vi "SAVE_DATA.vi"(0 "Q_Process_Data_IN":refnum<queue>, 1 "Q_Process_Data_Err_IN":errorcluster, 2 "Q_SEND_IN":refnum<queue>, 3 "Q_SEND_Err_IN":errorcluster, 4 "Notifier_IN":refnum<notifier>, 5 "Notifier_Error_IN":errorcluster, 6 "Q_Process_Data2_IN":refnum<queue>, 8 "Q_Process_Data2_Err_IN":errorcluster caption="error out") -> (16 "Q_SEND_OUT":refnum<queue>, 17 "Q_SEND_Err_OUT":errorcluster)   [LabVIEW 2019]
uses:
  <vilib>/Platform/TimedLoop/XDataNode/timing_clust.ctl
  <vilib>/Platform/TimedLoop/XDataNode/nitl_modes.ctl
  <vilib>/Platform/TimedLoop/XDataNode/wakeup.ctl
  Type/Type_TCP_Cmd.ctl
  RT_GLOBAL.vi
  <vilib>/Platform/TimedLoop/XDataNode/XDataNode.xnode
  <vilib>/Platform/TimedLoop/XDataNode/XDNodeRunTimeDep.lvlib
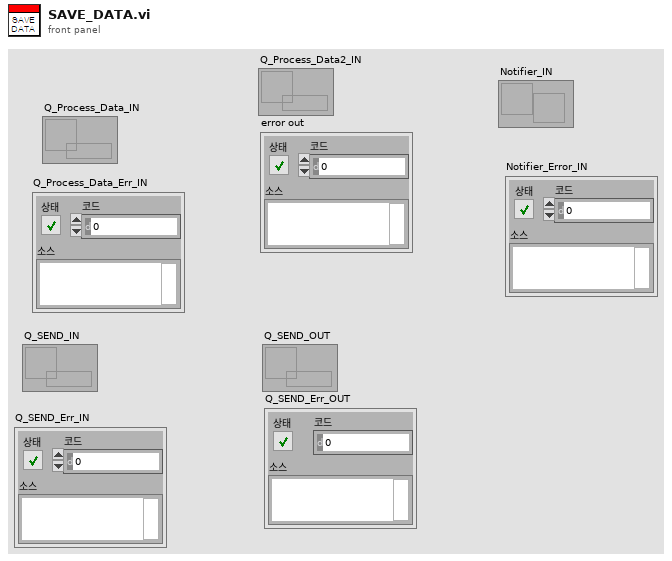
[diagram p1: front panel]
types:
  T1 = cluster{"Num_L":u32, "Period_L":u32, "GCP_L":sgl, "Num_R":u32, "Period_R":u32, "GCP_R":sgl, "FPGA_Data":sgl[], "Status_L":cluster{"Ready to switch on":bool, "Switched on":bool, "Operation enable":bool, "Fault":bool, "Voltage enable":bool, "Quick stop":bool, "Switch on disable":bool, "not used (warning)":bool, "Offset current measured":bool, "Remote":bool, "Operation mode specific":bool, "Internal limit active":bool, "Operation mode specific":bool, "Operation mode specific":bool, "Refresh cycle of power stage":bool, "Position referenced to home position":bool}, "Status_R":cluster{"Ready to switch on":bool, "Switched on":bool, "Operation enable":bool, "Fault":bool, "Voltage enable":bool, "Quick stop":bool, "Switch on disable":bool, "not used (warning)":bool, "Offset current measured":bool, "Remote":bool, "Operation mode specific":bool, "Internal limit active":bool, "Operation mode specific":bool, "Operation mode specific":bool, "Refresh cycle of power stage":bool, "Position referenced to home position":bool}, "Pos_L":i32, "Pos_R":i32, "TargetPos_L":i32, "TargetPos_R":i32, "Flag_L":enum16{"Release_Start", "Onset_Start", "Peak_Start", "Calculate"}, "Flag_R":enum16{"Release_Start", "Onset_Start", "Peak_Start", "Calculate"}, "LOAD_CELL_PEAK_L":sgl[], "LOAD_CELL_PEAK_R":sgl[], "D_Pos_L":i32, "D_Pos_R":i32, "A_Velocity_L":i32, "A_Velocity_R":i32, "A_Current_L":i16, "A_Current_R":i16}
  T2 = cluster{"Num_L":u32, "Period_L":u32, "GCP_L":sgl, "Num_R":u32, "Period_R":u32, "GCP_R":sgl, "FPGA_Data":sgl[], "Status_L":cluster{"Ready to switch on":bool, "Switched on":bool, "Operation enable":bool, "Fault":bool, "Voltage enable":bool, "Quick stop":bool, "Switch on disable":bool, "not used (warning)":bool, "Offset current measured":bool, "Remote":bool, "Operation mode specific":bool, "Internal limit active":bool, "Operation mode specific":bool, "Operation mode specific":bool, "Refresh cycle of power stage":bool, "Position referenced to home position":bool}, "Status_R":cluster{"Ready to switch on":bool, "Switched on":bool, "Operation enable":bool, "Fault":bool, "Voltage enable":bool, "Quick stop":bool, "Switch on disable":bool, "not used (warning)":bool, "Offset current measured":bool, "Remote":bool, "Operation mode specific":bool, "Internal limit active":bool, "Operation mode specific":bool, "Operation mode specific":bool, "Refresh cycle of power stage":bool, "Position referenced to home position":bool}, "Pos_L":i32, "Pos_R":i32, "TargetPos_L":i32, "TargetPos_R":i32, "Flag_L":enum16{"Release_Start", "Onset_Start", "Peak_Start", "Calculate"}, "Flag_R":enum16{"Release_Start", "Onset_Start", "Peak_Start", "Calculate"}, "LOAD_CELL_PEAK_L":sgl[], "LOAD_CELL_PEAK_R":sgl[], "D_Pos_L":i32, "D_Pos_R":i32, "A_Velocity_L":i32, "A_Velocity_R":i32, "A_Current_L":i16, "A_Current_R":i16}[]
  T3 = typedef "XDNodeRunTimeDep.lvlib/timing_clust.ctl" = cluster{"Expected End [f-1]":u64, "Actual End [f-1]":u64, "Finished Late? [f-1]":bool, "Expected End [i-1]":u64, "Actual End [i-1]":u64, "Finished Late? [i-1]":bool, "Expected Start [i]":u64, "Actual Start [i]":u64, "Expected Start [f]":u64, "Actual Start [f]":u64, "Source Name":string, "Structure Name":string, "Period":i64, "Deadline":i64, "Offset":i64, "Start":i64, "Priority":i32, "Timeout":i32, "Mode":T4, "Wakeup Reason":T5, "Error":errorcluster, "Source Type":string, "Secondary Source Type":string, "Global End Time":u64, "Global Start Time":u64, "Frame Duration":u64, "Iteration Duration":u64, "Assigned CPU":i32, "I/O Scan Engine Mode":u32}
  T4 = typedef "XDNodeRunTimeDep.lvlib/nitl_modes.ctl" = enum32{"No Change", "Process missed periods, maintain original phase", "Discard missed periods, maintain original phase", "Process missed periods, ignore original phase", "Discard missed periods, ignore original phase"}
  T5 = typedef "XDNodeRunTimeDep.lvlib/wakeup.ctl" = enum32{"Normal", "Aborted", "Asynchronous wakeup", "Timing source error", "Timed loop error", "Timeout"}
  T6 = typedef "Type_TCP_Cmd.ctl" = enum16{"None", "Data", "Config", "Active"}
  T7 = enum16{"open", "replace", "create", "open or create", "replace or create", "replace or create with confirmation"}
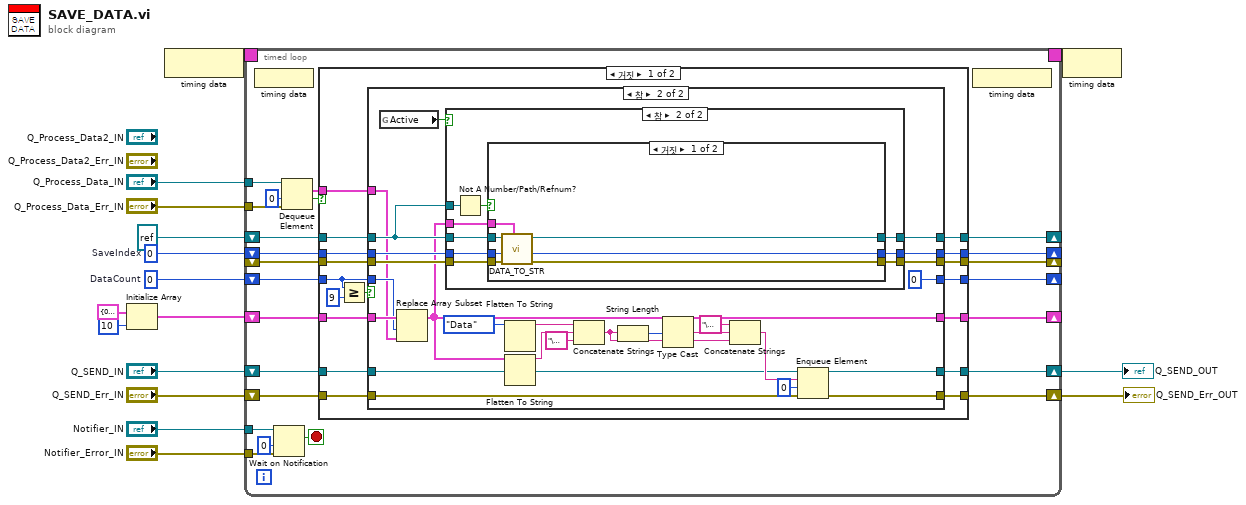
[diagram p0: block diagram]
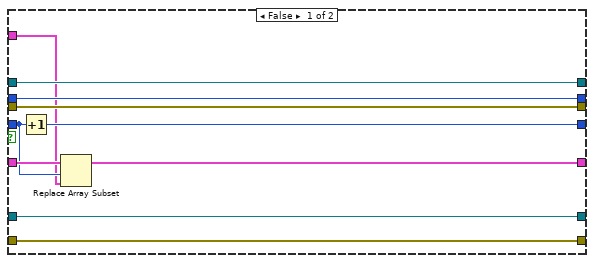
[diagram p2: hidden frame]
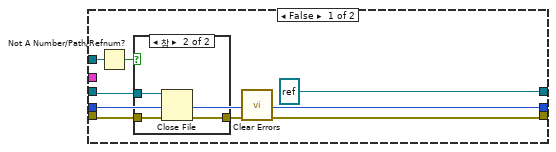
[diagram p3: hidden frame]
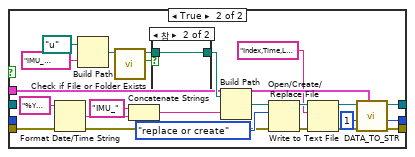
[diagram p5: hidden frame]
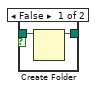
[diagram p6: hidden frame]
diagram:
  w14 = 0  # DataCount
  w15 = u32 0  # SaveIndex
  n1 = Initialize Array(T1 {"Num_L"=0, "Period_L"=0, "GCP_L"=0.0, "Num_R"=0, "Period_R"=0, "GCP_R"=0.0, "FPGA_Data"=[], "Status_L"={"Ready to switch on"=TRUE, "Switched on"=TRUE, "Operation enable"=TRUE, "Fault"=FALSE, "Voltage enable"=TRUE, "Quick stop"=TRUE, "Switch on disable"=FALSE, "not used (warning)"=FALSE, "Offset current measured"=FALSE, "Remote"=TRUE, "Operation mode specific"=TRUE, "Internal limit active"=FALSE, "Operation mode specific"=FALSE, "Operation mode specific"=FALSE, "Refresh cycle of power stage"=FALSE, "Position referenced to home position"=FALSE}, "Status_R"={"Ready to switch on"=TRUE, "Switched on"=TRUE, "Operation enable"=TRUE, "Fault"=FALSE, "Voltage enable"=TRUE, "Quick stop"=TRUE, "Switch on disable"=FALSE, "not used (warning)"=FALSE, "Offset current measured"=FALSE, "Remote"=TRUE, "Operation mode specific"=TRUE, "Internal limit active"=FALSE, "Operation mode specific"=FALSE, "Operation mode specific"=FALSE, "Refresh cycle of power stage"=FALSE, "Position referenced to home position"=FALSE}, "Pos_L"=0, "Pos_R"=0, "TargetPos_L"=0, "TargetPos_R"=0, "Flag_L"=enum."Release_Start", "Flag_R"=enum."Release_Start", "LOAD_CELL_PEAK_L"=[12.0, 8.0], "LOAD_CELL_PEAK_R"=[], "D_Pos_L"=0, "D_Pos_R"=0, "A_Velocity_L"=0, "A_Velocity_R"=0, "A_Current_L"=0, "A_Current_R"=0}, 10 ("차원 크기")) -> (w13:T2)
  n2 = node-c288() -> (w5:T3)
  n3 = timed-loop {
    tunnel: "Q_Process_Data_IN" -> [w38]
    tunnel: "Q_Process_Data_Err_IN" -> [w37]
    shift-right: [w34] -> _
    shift-left: refnum<file> refnum ("참조 번호 출력") -> [w35]
    shift-right: [w32] -> _
    shift-left: _ -> [w33]
    shift-right: [w31] -> _
    shift-left: w15 -> [w30]
    shift-right: [w28] -> _
    shift-left: w14 -> [w29]
    shift-right: [w26] -> _
    shift-left: w13 -> [w27]
    shift-right: [w24] -> w11
    shift-left: "Q_SEND_IN" -> [w25]
    shift-right: [w22] -> w10
    shift-left: "Q_SEND_Err_IN" -> [w23]
    timing: w5 -> [_]
    timing-out: [_] -> w4
    tunnel: "Notifier_IN" -> [w19]
    tunnel: "Notifier_Error_IN" -> [w18]
    stop <- w17 stop-if-true
    n4 = node-c288() -> ()  [unwired: 1 in]
    n5 = Wait on Notification(notifier=w19, timeout in ms (-1)=0 ("타임아웃(ms) (-1)"), error in (no error)=w18) -> (notification=w17:bool)  [unwired: 1 in, 3 out]
    n6 = Dequeue Element(queue=w38, timeout in ms (-1)=0 ("타임아웃(ms) (-1)"), error in (no error)=w37) -> (element=w36:T1, timed out?=w21:bool)  [unwired: 2 out]
    n7 = case shown="거짓" w21 {
      tunnel: w36 -> [w47 _]
      tunnel: w35 -> [w43 w155]
      tunnel: [w42 w155] -> w34
      tunnel: [w44 w154] -> w32
      tunnel: w33 -> [w45 w154]
      tunnel: [w49 w153] -> w31
      tunnel: w30 -> [w50 w153]
      tunnel: w29 -> [w52 w152]
      tunnel: [w51 w152] -> w28
      tunnel: w27 -> [w48 w151]
      tunnel: [w46 w151] -> w26
      tunnel: [w56 w150] -> w24
      tunnel: w25 -> [w58 w150]
      tunnel: [w55 w149] -> w22
      tunnel: w23 -> [w57 w149]
      frame False {
        n8 = Greater Or Equal?(x=w52, y=9) -> (x >= y?=w53:bool)
        n9 = case shown="참" w53 {
          tunnel: w58 -> [w68 w79]
          tunnel: w57 -> [w67 w77]
          tunnel: [w68 w78] -> w56
          tunnel: [w67 w76] -> w55
          tunnel: [w65 0] -> w51
          tunnel: w52 -> [w63 w93]
          tunnel: w50 -> [w66 w92]
          tunnel: [w66 w72] -> w49
          tunnel: w48 -> [w64 w94]
          tunnel: w47 -> [w59 w69]
          tunnel: [w62 w71] -> w46
          tunnel: [w61 w73] -> w44
          tunnel: w45 -> [w61 w91]
          tunnel: [w60 w74] -> w42
          tunnel: w43 -> [w60 w90]
          frame False {
            n10 = Increment(x=w63) -> (x+1=w65:i32)
            n11 = Replace Array Subset(array=w64, new element=w59, index=w63) -> (w62:T2)
          }
          frame True {
            n12 = global read "RT_GLOBAL.vi" "Active"() -> (w70:bool)
            n13 = Replace Array Subset(array=w94, new element=w69, index=w93) -> (w71:T2)
            n14 = case shown="참" w70 {
              tunnel: w92 -> [w95 w111]
              tunnel: w91 -> [w100 w113]
              tunnel: w90 -> [w99 w112]
              tunnel: w90 -> [w98 w115]
              tunnel: [refnum<file> refnum ("참조 번호 출력") w110] -> w74
              tunnel: [w96 w109] -> w73
              tunnel: [w95 w108] -> w72
              tunnel: w71 -> [_ w107]
              frame False {
                n15 = Not A Number/Path/Refnum?(number/path/refnum=w98) -> (NaN/Path/Refnum?=w102:bool)
                n16 = case shown="참" w102 {
                  tunnel: w99 -> [_ w106]
                  tunnel: w100 -> [w103 w105]
                  tunnel: [w103 w104] -> w101
                  frame False {
                  }
                  frame True {
                    n17 = Close File(refnum=w106, error in=w105) -> (error out=w104:errorcluster)  [unwired: 1 out]
                  }
                }
                n18 = call <vilib>:"Clear Errors.vi"("error in (no error)"=w101) -> ("error out"=w96:errorcluster)  [unwired: 5 in, 1 out]
              }
              frame True {
                n19 = Not A Number/Path/Refnum?(number/path/refnum=w115) -> (NaN/Path/Refnum?=w114:bool)
                n20 = case shown="거짓" w114 {
                  tunnel: w113 -> [w122 w129]
                  tunnel: w112 -> [w120 _]
                  tunnel: w111 -> [w121 _]
                  tunnel: [w119 w126] -> w110
                  tunnel: [w118 w127] -> w109
                  tunnel: [w117 w125] -> w108
                  tunnel: w107 -> [w116 w128]
                  frame False {
                    n21 = call "DATA_TO_STR.vi"("DATA"=w116, "ref_File_ErrIn"=w122, "Index"=w121, "ref_File_In"=w120) -> ("ref_File_ErrOut"=w118:errorcluster, "Index_Out"=w117:u32, "ref_File_Out"=w119:refnum<file>)  [unwired: 5 in]
                  }
                  frame True {
                    n22 = Format Date/Time String(time format string (%c)="%Y%m%d_%H%M%S.csv" ("시간 포맷 문자열 (%c)")) -> (date/time string=w140:string)  [unwired: 2 in]
                    n23 = Build Path(base path=path "u:/" ("베이스 경로"), name or relative path="IMU_SENSOR" ("시간 포맷 문자열 (%c)")) -> (appended path=w145:path)
                    n24 = call <vilib>:"Check if File or Folder Exists.vi"("path"=w145) -> ("file or folder exists?"=w144:bool, "dup path"=w143:path)  [unwired: 8 in, 1 out]
                    n25 = Concatenate Strings("IMU_" ("문자열"), w140) -> (w141:string)
                    n26 = case shown="참" w144 {
                      tunnel: w143 -> [w147 w148]
                      tunnel: [w146 w148] -> w142
                      frame False {
                        n27 = Create Folder(path (use dialog)=w147) -> (created path=w146:path)  [unwired: 2 in, 2 out]
                      }
                      frame True {
                      }
                    }
                    n28 = Build Path(base path=w142, name or relative path=w141) -> (appended path=w136:path)
                    n29 = Open/Create/Replace File(file path (use dialog)=w136, error in=w129, operation (0:open)=T7."replace or create" ("동작(0:open)")) -> (refnum out=w135:refnum<file>, error out=w134:errorcluster)  [unwired: 3 in, 1 out]
                    n30 = Write to Text File(file (use dialog)=w135, text="Index,Time,L_Load,R_Load,L_Roll,L_Pitch,L_Yaw,L_accX,L_accY,L_accZ,R_Roll,R_Pitch,R_Yaw,R_accX,R_accY,R_accZ,L_Flag,R_Flag,L_GCP,R_GCP,L_Pos,R_Pos,L_TargetPos,R_TargetPos,MaxLoad_L,OnsetLoad_L,MaxLoad_R,OnsetLoad_R,D_Pos_L,D_Pos_R,A_Velocity_L,A_Velocity_R,A_Current_L,A_Current_R,B_Roll,B_Pitch,B_Yaw,B_accX,B_accY,B_accZ\n" ("텍스트"), error in=w134) -> (refnum out=w132:refnum<file>, error out=w131:errorcluster)  [unwired: 1 in, 1 out]
                    n31 = call "DATA_TO_STR.vi"("DATA"=w128, "ref_File_ErrIn"=w131, "Index"=u32 1, "ref_File_In"=w132) -> ("ref_File_ErrOut"=w127:errorcluster, "Index_Out"=w125:u32, "ref_File_Out"=w126:refnum<file>)  [unwired: 5 in]
                  }
                }
              }
            }
            n32 = Flatten To String(anything=Type_TCP_Cmd."Data") -> (data string=w84:string)  [unwired: 3 in, 2 out]
            n33 = Flatten To String(anything=w71) -> (data string=w85:string)  [unwired: 3 in, 2 out]
            n34 = Concatenate Strings(w84, w85, "\u0003" ("문자열")) -> (w82:string)
            n35 = String Length(string=w82) -> (length=w86:i32)
            n36 = Type Cast(x=w86) -> (*(type *) &x=w87:string)  [unwired: 1 in]
            n37 = Concatenate Strings("\u0002" ("문자열"), w87, w82) -> (w80:string)
            n38 = Enqueue Element(queue=w79, element=w80, timeout in ms (-1)=0 ("타임아웃(ms) (-1)"), error in (no error)=w77) -> (queue out=w78:refnum<queue>, error out=w76:errorcluster)  [unwired: 1 out]
          }
        }
      }
      frame True {
      }
    }
    n39 = node-c288() -> ()  [unwired: 1 out]
  }
  "Q_SEND_OUT" <- w11
  "Q_SEND_Err_OUT" <- w10
  n40 = node-c288(w4) -> ()
